vi "Init Winch Spark Max With CVS File.vi"(3 "error in":errorcluster, 4 "Motor ID":string="Winch", 5 "Robot ID":string="981") -> (0 "error out":errorcluster, 1 "Can Bus ID":u8, 2 "CAN Talon SRX Ref":T1={"DeviceStatus"={"status"=FALSE, "code"=0, "source"=""}, "Type"=enum."PWM", "PWM"={"PWM Channel"=enum."PWM 1", "DeadBand"={"Name"="", "maxPositivePwm"=0, "minPositivePwm"=0, "centerPwm"=0, "maxNegativePwm"=0, "minNegativePwm"=0, "angularRange"=0}}, "CAN"={"Device Number"=0, "SetOutput VI Ref"=variant(enum8{"Percent VBus", "Current", "Speed", "Position", "Voltage"} enum."Percent VBus"), "GetOutput VI Ref"=variant(refnum<k1> refnum), "Enable VI Ref"=variant(dbl 12.0), "Disable VI Ref"=variant(enum8{"Percent VBus", "Speed", "Position", "Slave", "Unchanged / Invalid", "Voltage Compensation", "Current", "Motion Profile"} enum."Percent VBus"), "Data"=variant}, "Invert"=FALSE, "DIO PWM"={"PWM \"Enable\" Channel"=enum."Invalid", "DIOChannel"=enum."Invalid", "PWM Rate"=0.0}})   [LabVIEW 2020]
uses:
  <vilib>/Rock Robotics/WPI/MotorControl/WPI_MotorControlDeviceRef.ctl
  <vilib>/Rock Robotics/WPI/MotorControl/WPI_MotorControlType.ctl
  <vilib>/Rock Robotics/SystemInterfaces/DIO/FPGA_DIOPWMChannel.ctl
  <vilib>/Rock Robotics/WPI/PWM/WPI_PWMDeadband.ctl
  <vilib>/Rock Robotics/SystemInterfaces/DIO/FPGA_DIOChannel.ctl
  2022 Robot Global Data.vi
panel:
  out "Can Motor ID":u8
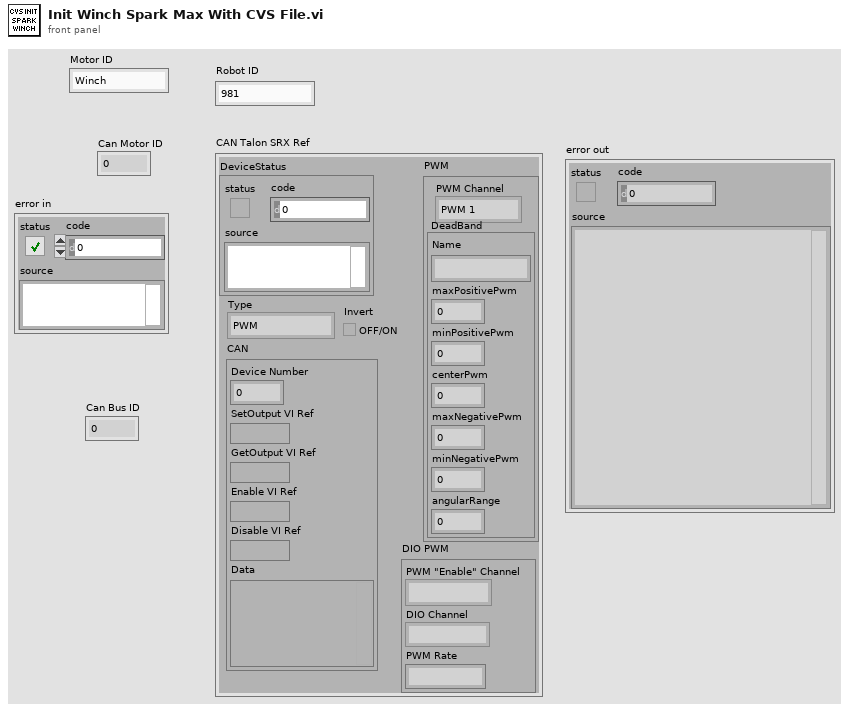
[diagram p1: front panel]
types:
  T1 = typedef "WPI_MotorControlDeviceRef.ctl" = cluster{"DeviceStatus":errorcluster, "Type":T2, "PWM":cluster{"PWM Channel":T3, "DeadBand":T4}, "CAN":cluster{"Device Number":u8, "SetOutput VI Ref":variant, "GetOutput VI Ref":variant, "Enable VI Ref":variant, "Disable VI Ref":variant, "Data":variant}, "Invert":bool, "DIO PWM":cluster{"PWM \"Enable\" Channel":T3, "DIOChannel":T5, "PWM Rate":dbl}}
  T2 = typedef "WPI_MotorControlType.ctl" = enum16{"PWM", "CAN", "DIO PWM"}
  T3 = typedef "FPGA_DIOPWMChannel.ctl" = enum8{"PWM 0", "PWM 1", "PWM 2", "PWM 3", "PWM 4", "PWM 5", "PWM 6", "PWM 7", "PWM 8", "PWM 9", "PWM MXP 0", "PWM MXP 1", "PWM MXP 2", "PWM MXP 3", "PWM MXP 4", "PWM MXP 5", "PWM MXP 6", "PWM MXP 7", "PWM MXP 8", "PWM MXP 9", "Invalid"}
  T4 = typedef "WPI_PWMDeadband.ctl" = cluster{"Name":string, "maxPositivePwm":i32, "minPositivePwm":i32, "centerPwm":i32, "maxNegativePwm":i32, "minNegativePwm":i32, "angularRange":u16}
  T5 = typedef "FPGA_DIOChannel.ctl" = enum8{"DIO 0", "DIO 1", "DIO 2", "DIO 3", "DIO 4", "DIO 5", "DIO 6", "DIO 7", "DIO 8", "DIO 9", "DIO MXP 0", "DIO MXP 1", "DIO MXP 2", "DIO MXP 3", "DIO MXP 4", "DIO MXP 5", "DIO MXP 6", "DIO MXP 7", "DIO MXP 8", "DIO MXP 9", "DIO MXP 10", "DIO MXP 11", "DIO MXP 12", "DIO MXP 13", "DIO MXP 14", "DIO MXP 15", "SPI Port CS1", "SPI Port CS2", "SPI Port CS3", "SPI Port MISO", "SPI Port MOSI", "Invalid"}
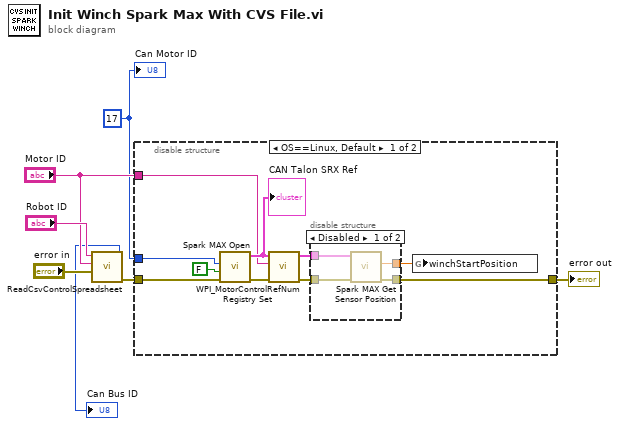
[diagram p0: block diagram]
diagram:
  w2 = u8 17 ("Can Motor ID")
  n1 = call "ReadCsvControlSpreadsheet.vi"("error in"="error in", "Motor ID"="Motor ID", "Robot ID"="Robot ID") -> ("error out"=w5:errorcluster, "Can Bus ID"=→"Can Bus ID":u8)  [unwired: 7 out]
  n2 = disable-structure shown="OS==Linux, Default" {
    disable-tunnel: "Motor ID" -> [w13 _]
    disable-tunnel: w5 -> [w17 w22]
    disable-tunnel: [w9 w22] -> w4
    disable-tunnel: w2 -> [w16 _]
    frame condition #0 (active) {
      n3 = call <vilib>:"Spark MAX Open.vi"("error in (no error)"=w17, "Invert"=FALSE, "Device Number"=w16) -> ("error out"=w15:errorcluster, "MotorControlDeviceRef"=w14:T1)  [unwired: 7 in]
      "CAN Talon SRX Ref" <- w14
      n4 = call <vilib>:"WPI_MotorControlRefNum Registry Set.vi"("error in (no error)"=w15, "refnum name"=w13, "MotorControlDevRef"=w14) -> ("error out"=w10:errorcluster, "MotorControlDevRef"=w11:T1)  [unwired: 7 in]
      n5 = disable-structure shown="Disabled" {
        disable-tunnel: w11 -> [w21 _]
        disable-tunnel: w10 -> [w20 _]
        disable-tunnel: [w19 _] -> w9
        disable-tunnel: [w18 _] -> w8
        frame Disabled {
          n6 = call <vilib>:"Spark MAX Get Sensor Position.vi"("error in (no error)"=w20, "MotorControlDevRef in"=w21) -> ("error out"=w19:errorcluster, "Sensor Position"=w18:dbl)  [unwired: 6 in, 2 out]
        }
        frame Enabled {
        }
      }
      n7 = global write "2022 Robot Global Data.vi" "winchStartPosition"(w8) -> ()
    }
    frame condition #1 {
    }
  }
  "error out" <- w4
  "Can Motor ID" <- w2
